vi "ZeroStatus.vi"(0 "VisaCluster":T1, 11 "error in (no error)":errorcluster) -> (4 "VisaCluster":T1, 8 "Answer":string, 15 "error out":errorcluster)   [LabVIEW 2014, in "FH 55.lvlib"]
uses:
  FH 55.lvlib
  TypeDef/VisaCluster.ctl
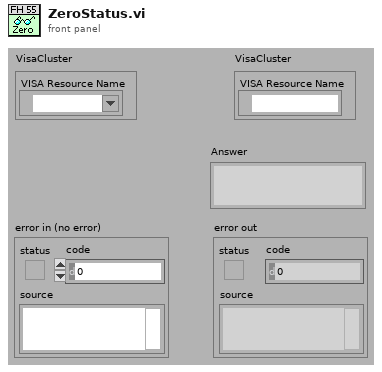
[diagram p1: front panel]
types:
  T1 = typedef "FH 55.lvlib/VisaCluster.ctl" = cluster{"VISA Resource Name":refnum<visa-resource-name>}
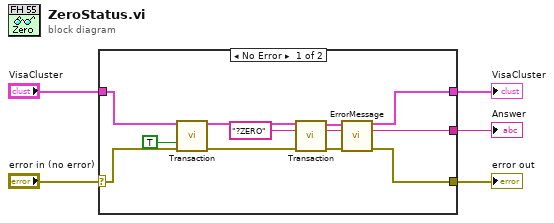
[diagram p0: block diagram]
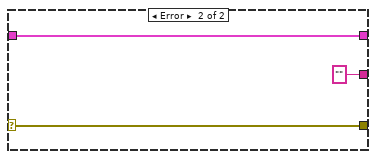
[diagram p2: hidden frame]
diagram:
  n1 = case shown="No Error" "error in (no error)" {
    selector: "error in (no error)" -> [w13 w19]
    tunnel: "VisaCluster" -> [w11 w20]
    tunnel: [w17 w20] -> w1
    tunnel: [w7 w19] -> w3
    tunnel: [w6 ""] -> w2
    frame No Error {
      n2 = call "Transaction.vi"("VisaCluster"=w11, "Read Only? (False)"=TRUE, "error in (no error)"=w13) -> ("VisaCluster"=w10:T1, "error out"=w12:errorcluster)  [unwired: 9 in, 2 out]
      n3 = call "Transaction.vi"("VisaCluster"=w10, "Command"="?ZERO", "error in (no error)"=w12) -> ("VisaCluster"=w15:T1, "Answer"=w8:string, "error out"=w16:errorcluster)  [unwired: 9 in, 1 out]
      n4 = call "ErrorMessage.vi"("VisaCluster"=w15, "Message In"=w8, "error in (no error)"=w16) -> ("VisaCluster"=w17:T1, "Message Out"=w6:string, "error out"=w7:errorcluster)  [unwired: 10 in]
    }
    frame Error {
    }
  }
  "error out" <- w3
  "Answer" <- w2
  "VisaCluster" <- w1
